vi "ANC300_Close.vi"(0 "ANC300 Communication Port In":refnum<visa-resource-name>, 1 "connection ID in":refnum<k5>, 5 "error in":T1) -> (19 "error out":T1)   [LabVIEW 2022 SP3]
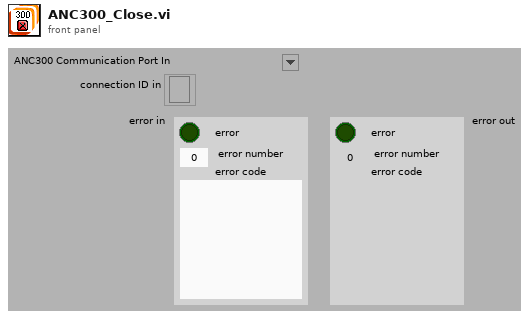
[diagram p1: front panel]
types:
  T1 = cluster{"error ":bool, "error number":i32, "error code":string}
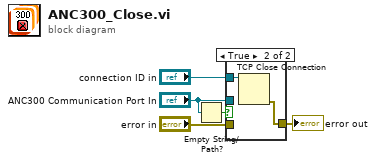
[diagram p0: block diagram]
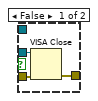
[diagram p2: hidden frame]
diagram:
  n1 = Empty String/Path?(string/path="ANC300 Communication Port In") -> (empty?=w2:bool)
  n2 = case shown="True" w2 {
    tunnel: [w8 w9] -> w5
    tunnel: "ANC300 Communication Port In" -> [w7 _]
    tunnel: "error in" -> [w6 _]
    tunnel: "connection ID in" -> [_ w10]
    frame False {
      n3 = VISA Close(VISA resource name=w7, error in (no error)=w6) -> (error out=w8:errorcluster)
    }
    frame True {
      n4 = TCP Close Connection(connection ID=w10) -> (error out=w9:errorcluster)  [unwired: 2 in, 1 out]
    }
  }
  "error out" <- w5
